vi "test.vi"() -> ()   [LabVIEW 2017]
uses:
  <vilib>/addons/database/Connection.llb/DB Tools Open Connec (Path).vi
  <vilib>/addons/database/NI_Database_API.lvlib
panel:
  in  "Stakeholder":string(combo)
  out "Array":string[][](array[string])
  in  "Station":string(combo)
  in  "Shift":string(combo)
  in  "To Date":timestamp format="%<%Y-%m-%d>T"
  in  "From Date":timestamp format="%<%Y-%m-%d>T"
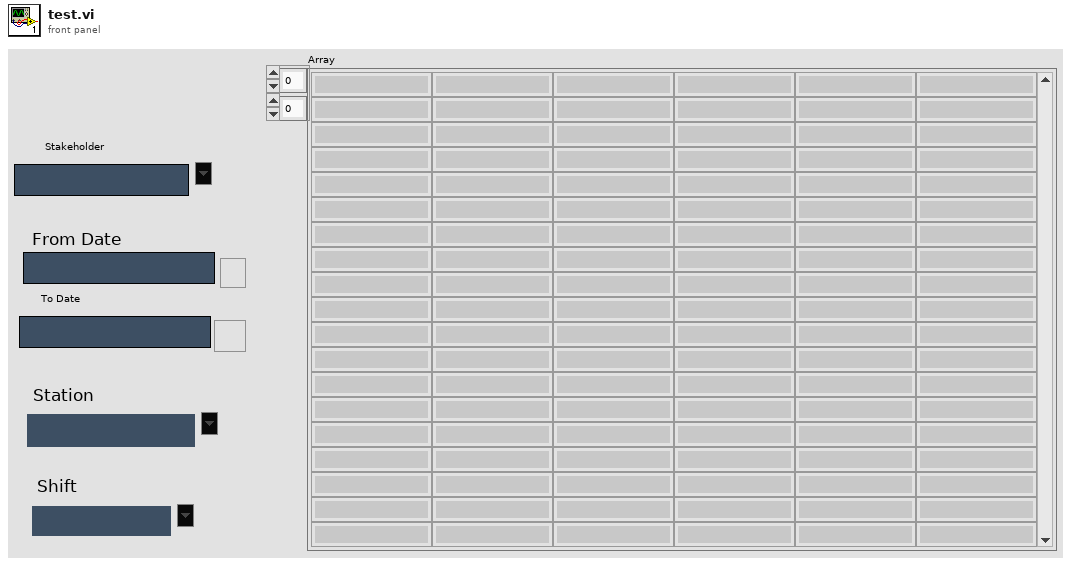
[diagram p1: front panel]
types:
  T1 = typedef "NI_Database_API.lvlib/Conn ObjectReference.ctl" = refnum<k1>
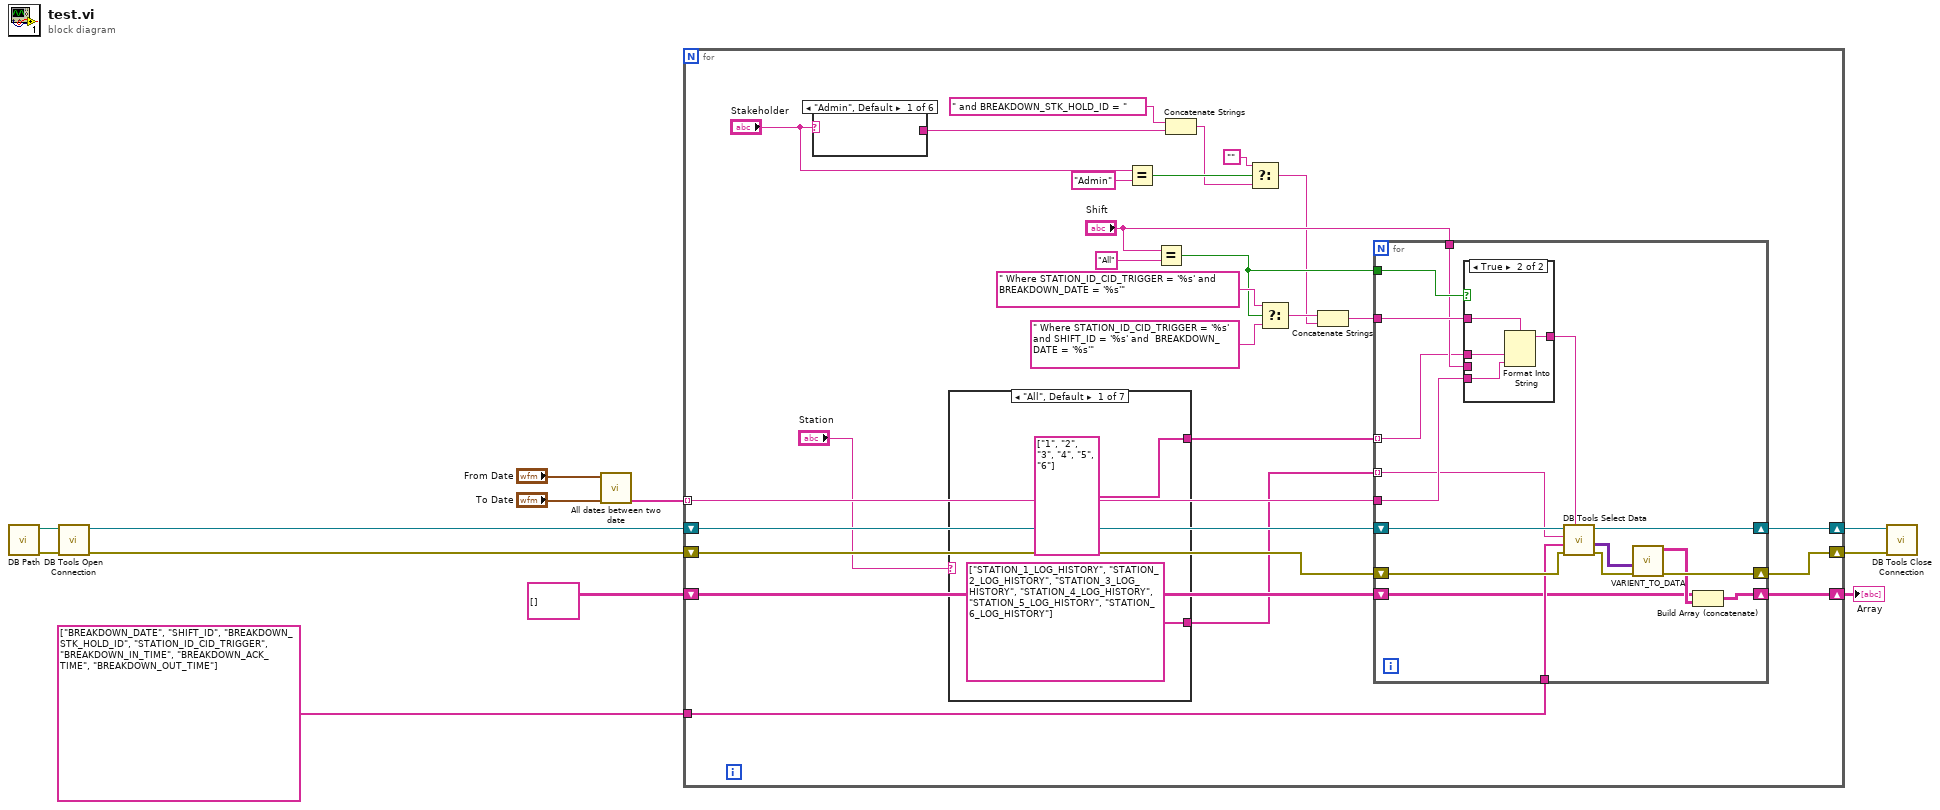
[diagram p0: block diagram]
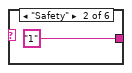
[diagram p2: hidden frame]
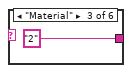
[diagram p3: hidden frame]
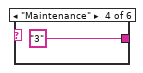
[diagram p4: hidden frame]
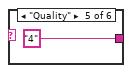
[diagram p5: hidden frame]
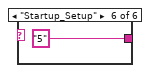
[diagram p6: hidden frame]
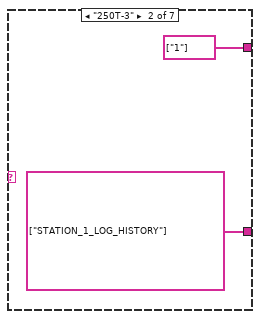
[diagram p7: hidden frame]
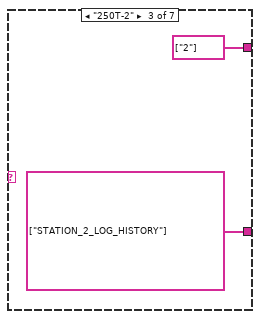
[diagram p8: hidden frame]
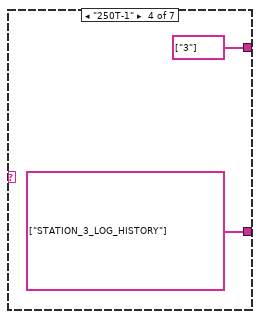
[diagram p9: hidden frame]
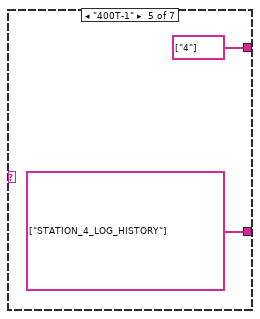
[diagram p10: hidden frame]
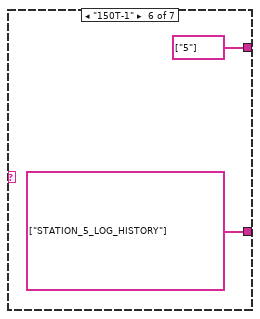
[diagram p11: hidden frame]
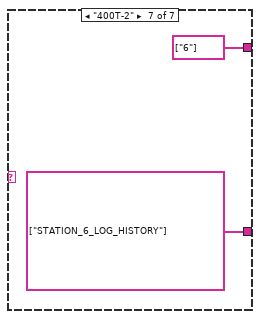
[diagram p12: hidden frame]
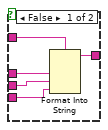
[diagram p13: hidden frame]
diagram:
  n1 = call "DB Path.vi"() -> ("error out"=w12:errorcluster, "DB Path"=w11:path)  [unwired: 10 in]
  n2 = call-poly <vilib>:"DB Tools Open Connection.vi"("error in (no error)"=w12, "connection information"=w11) -> ("error out"=w9:errorcluster, "connection reference"=w10:T1)  [unwired: 6 in]
  n3 = call "All dates between two date.vi"("To Date"="To Date", "From Date"="From Date") -> ("All Days (String)"=w1:string[])  [unwired: 8 in, 1 out]
  n4 = for {
    tunnel: string[] ["BREAKDOWN_DATE", "SHIFT_ID", "BREAKDOWN_STK_HOLD_ID", "STATION_ID_CID_TRIGGER", "BREAKDOWN_IN_TIME", "BREAKDOWN_ACK_TIME", "BREAKDOWN_OUT_TIME"] -> [w36]
    shift-right: [w30] -> w5
    shift-left: w10 -> [w38]
    shift-right: [w29] -> w4
    shift-left: w9 -> [w37]
    shift-right: [w27] -> w6
    shift-left: string[][] [] -> [w28]
    tunnel: w1 -> [w26] mode=indexing
    n5 = case shown="\"Admin\", Default" "Stakeholder" {
      tunnel: [_ "1" "2" "3" "4" "5"] -> w18
      frame "Admin", Default {
      }
      frame "Safety" {
      }
      frame "Material" {
      }
      frame "Maintenance" {
      }
      frame "Quality" {
      }
      frame "Startup_Setup" {
      }
    }
    n6 = case shown="\"All\", Default" "Station" {
      tunnel: [string[] ["STATION_1_LOG_HISTORY", "STATION_2_LOG_HISTORY", "STATION_3_LOG_HISTORY", "STATION_4_LOG_HISTORY", "STATION_5_LOG_HISTORY", "STATION_6_LOG_HISTORY"] string[] ["STATION_1_LOG_HISTORY"] string[] ["STATION_2_LOG_HISTORY"] string[] ["STATION_3_LOG_HISTORY"] string[] ["STATION_4_LOG_HISTORY"] string[] ["STATION_5_LOG_HISTORY"] string[] ["STATION_6_LOG_HISTORY"]] -> w24
      tunnel: [string[] ["1", "2", "3", "4", "5", "6"] string[] ["1"] string[] ["2"] string[] ["3"] string[] ["4"] string[] ["5"] string[] ["6"]] -> w23
      frame "All", Default {
      }
      frame "250T-3" {
      }
      frame "250T-2" {
      }
      frame "250T-1" {
      }
      frame "400T-1" {
      }
      frame "150T-1" {
      }
      frame "400T-2" {
      }
    }
    n7 = Equal?(x="Stakeholder", y="Admin") -> (x = y?=w21:bool)
    n8 = Equal?(x="Shift", y="All" ("x")) -> (x = y?=w32:bool)
    n9 = Concatenate Strings(" and BREAKDOWN_STK_HOLD_ID = " ("format string"), w18) -> (w17:string)
    n10 = Select(t="", s=w21, f=w17) -> (s? t:f=w14:string)
    n11 = Select(t=" Where STATION_ID_CID_TRIGGER = '%s' and BREAKDOWN_DATE = '%s'" ("format string"), s=w32, f=" Where STATION_ID_CID_TRIGGER = '%s' and SHIFT_ID = '%s' and  BREAKDOWN_DATE = '%s'" ("format string")) -> (s? t:f=w15:string)
    n12 = Concatenate Strings(w15, w14) -> (w13:string)
    n13 = for {
      tunnel: w36 -> [w72]
      tunnel: w26 -> [w66]
      tunnel: w13 -> [w69]
      tunnel: w32 -> [w68]
      tunnel: w24 -> [w59] mode=indexing
      tunnel: "Shift" -> [w67]
      shift-right: [w64] -> w29
      shift-left: w37 -> [w73]
      shift-right: [w63] -> w30
      shift-left: w38 -> [w74]
      shift-right: [w60] -> w27
      shift-left: w28 -> [w61]
      tunnel: w23 -> [w58] mode=indexing
      n14 = case shown="True" w68 {
        tunnel: w69 -> [w79 w83]
        tunnel: w58 -> [w78 w82]
        tunnel: w67 -> [w76 _]
        tunnel: w66 -> [w75 w80]
        tunnel: [w77 w81] -> w65
        frame False {
          n15 = Format Into String(format string=w79, w78, w76, w75) -> (resulting string=w77:string)  [unwired: 2 in, 1 out]
        }
        frame True {
          n16 = Format Into String(format string=w83, w82, w80) -> (resulting string=w81:string)  [unwired: 2 in, 1 out]
        }
      }
      n17 = call <vilib>:"DB Tools Select Data.vi"("condition"=w65, "error in (no error)"=w73, "columns"=w72, "table"=w59, "connection reference"=w74) -> ("error out"=w70:errorcluster, "data"=w71:variant[][], "connection reference out"=w63:T1)  [unwired: 1 in]
      n18 = call "VARIENT_TO_DATA.vi"("data"=w71, "error in (no error)"=w70) -> ("Table"=w62:string[][], "error out"=w64:errorcluster)  [unwired: 7 in]
      n19 = Build Array (concatenate)(w61, w62) -> (w60:string[][])
    }
  }
  "Array" <- w6
  n20 = call <vilib>:"DB Tools Close Connection.vi"("error in (no error)"=w4, "connection reference"=w5) -> ()  [unwired: 5 in, 1 out]
